vi "getFromDisplay.vi"(8 "error in (no error)":errorcluster, 11 "WinX32Settings in":refnum<class "WinX32Settings.lvclass">) -> (0 "error out":errorcluster, 3 "WinX32Settings out":refnum<class "WinX32Settings.lvclass">)   [LabVIEW 2011, in "Tools.lvlib" / "Settings.lvlib" / "WinX32Settings.lvclass"]
uses:
  WinX32Settings.lvclass
  WinX32Settings.lvclass/WinX32Settings.ctl
  CamaraSettings.lvclass
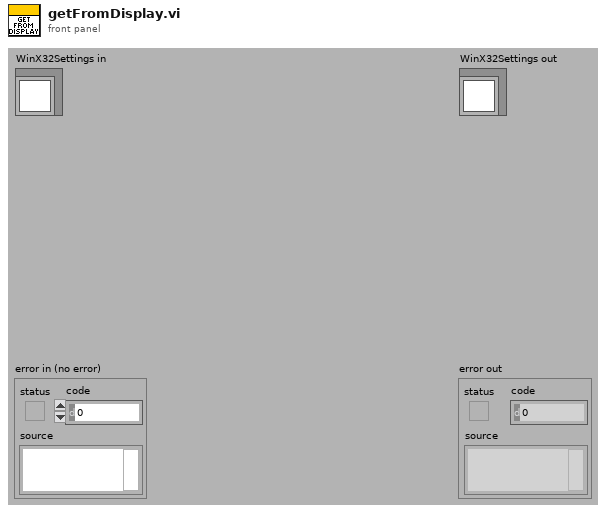
[diagram p1: front panel]
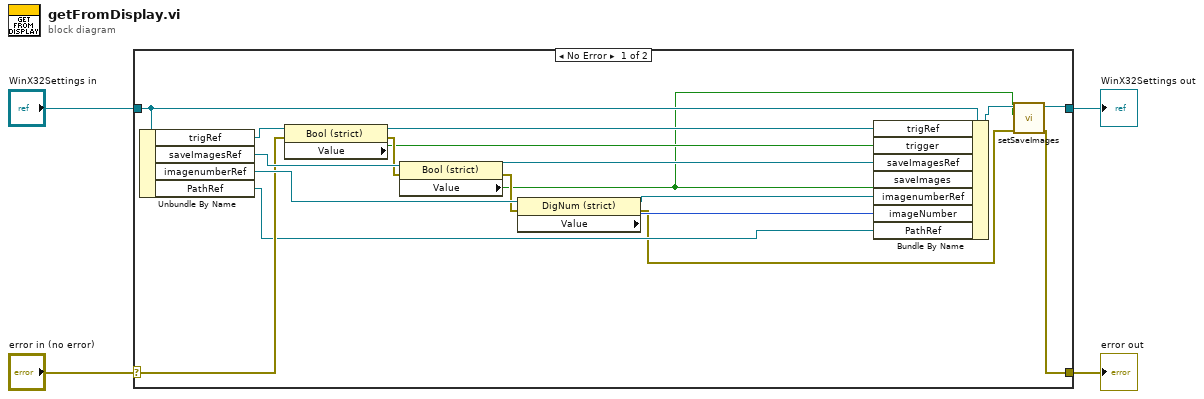
[diagram p0: block diagram]
diagram:
  n1 = case shown="No Error" "error in (no error)" {
    selector: "error in (no error)" -> [w12 w24]
    tunnel: [w8 w24] -> w3
    tunnel: [w7 w23] -> w1
    tunnel: "WinX32Settings in" -> [w11 w23]
    frame No Error {
      n2 = Unbundle By Name(w11) -> ("trigRef"=w22:refnum<vi>, "saveImagesRef"=w21:refnum<vi>, "imagenumberRef"=w20:refnum<vi>, "PathRef"=w6:refnum<vi>)
      n3 = property class="Bool (strict)"(reference=w22, error in=w12) -> (reference out=w17:refnum<vi>, error out=w19:errorcluster, "Value"=w16:bool)
      n4 = property class="Bool (strict)"(reference=w21, error in=w19) -> (reference out=w15:refnum<vi>, error out=w18:errorcluster, "Value"=w9:bool)
      n5 = property class="DigNum (strict)"(reference=w20, error in=w18) -> (reference out=w14:refnum<vi>, error out=w5:errorcluster, "Value"=w13:i32)
      n6 = Bundle By Name(cluster=w11, "trigRef"=w17, "trigger"=w16, "saveImagesRef"=w15, "saveImages"=w9, "imagenumberRef"=w14, "imageNumber"=w13, "PathRef"=w6) -> (w10:refnum<class "WinX32Settings.lvclass">)
      n7 = call "setSaveImages.vi"("error in (no error)"=w5, "saveImages"=w9, "CamaraSettings in"=w10) -> ("error out"=w8:errorcluster, "CamaraSettings out"=w7:refnum<class "WinX32Settings.lvclass">)  [unwired: 7 in]
    }
    frame Error {
    }
  }
  "error out" <- w3
  "WinX32Settings out" <- w1
